vi "Get Communication Line.vi"(8 "error in (no error)":errorcluster, 10 "Wavelength":u16, 11 "Laser Quantum in":refnum<class "Laser.lvclass">) -> (0 "error out":errorcluster, 1 "Laser Type":T1(ring), 2 "Serial Port":refnum<visa-resource-name>, 3 "Laser Quantum out":refnum<class "Laser.lvclass">, 4 "Polarizer Theta Zero":dbl, 6 "Polarizer Amplitude":dbl)   [LabVIEW 2018, in "Laser.lvlib" / "Laser.lvclass"]
uses:
  Laser.lvclass
  Laser.lvclass/Laser.ctl
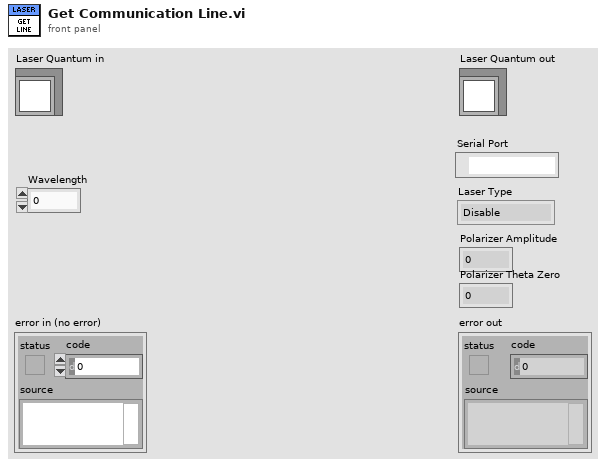
[diagram p1: front panel]
types:
  T1 = enum16{"Disable", "Laser Quantum", "Coherent OBIS", "PRM1-Z8", "Coherent HOPS"}
  T2 = enum16{"Disable", "Laser Quantum", "Coherent OBIS"}
  T3 = typedef "Laser Configuration.ctl" = cluster{"Serial Port":refnum<visa-resource-name>, "Laser Type":enum16{"Disable", "Laser Quantum", "Coherent OBIS", "PRM1-Z8", "Coherent HOPS"}, "Polarizer Amplitude":dbl, "Polarizer Theta Zero":dbl, "Wavelength":u16}
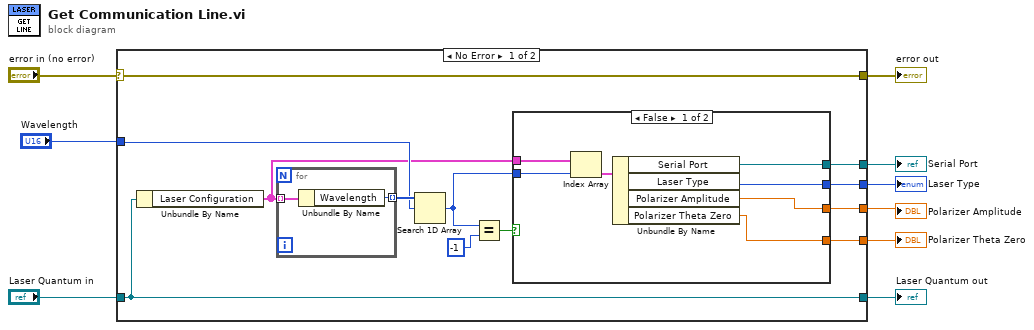
[diagram p0: block diagram]
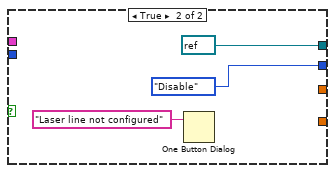
[diagram p2: hidden frame]
diagram:
  n1 = case shown="No Error" "error in (no error)" {
    selector: "error in (no error)" -> [w21 w35]
    tunnel: [w21 w35] -> w7
    tunnel: [w17 w34] -> w6
    tunnel: "Laser Quantum in" -> [w17 w34]
    tunnel: "Wavelength" -> [w19 _]
    tunnel: [w18 _] -> w5
    tunnel: [w15 _] -> w4
    tunnel: [w11 _] -> w3
    tunnel: [w10 _] -> w2
    frame No Error {
      n2 = Unbundle By Name(w17) -> ("Laser Configuration"=w16:T3[])
      n3 = for {
        tunnel: w16 -> [w33] mode=indexing
        tunnel: [w32] -> w20 mode=indexing
        n4 = Unbundle By Name(w33) -> ("Wavelength"=w32:u16)
      }
      n5 = Search 1D Array(1D array=w20, element=w19) -> (index of element=w13:i32)  [unwired: 1 in]
      n6 = Equal?(x=w13, y=-1) -> (x = y?=w14:bool)
      n7 = case shown="False" w14 {
        tunnel: [w28 refnum<visa-resource-name> refnum ("Serial Port")] -> w18
        tunnel: w13 -> [w27 _]
        tunnel: w16 -> [w26 _]
        tunnel: [w24 T2."Disable" ("Laser Type")] -> w15
        tunnel: [w23 _] -> w11
        tunnel: [w22 _] -> w10
        frame False {
          n8 = Index Array(array=w26, index=w27) -> (element=w25:T3)
          n9 = Unbundle By Name(w25) -> ("Serial Port"=w28:refnum<visa-resource-name>, "Laser Type"=w24:T1, "Polarizer Amplitude"=w23:dbl, "Polarizer Theta Zero"=w22:dbl)
        }
        frame True {
          n10 = One Button Dialog(message="Laser line not configured") -> ()  [unwired: 1 in, 1 out]
        }
      }
    }
    frame Error {
    }
  }
  "error out" <- w7
  "Laser Quantum out" <- w6
  "Serial Port" <- w5
  "Laser Type" <- w4
  "Polarizer Amplitude" <- w3
  "Polarizer Theta Zero" <- w2
